vi "FlatToRichniswitch_grpc_RouteScanAdvancedOutputRequest.vi"(5 "OutputClusterType":T1, 11 "InputCluster":T3) -> (3 "OutputCluster":T1)   [LabVIEW 2021, in "NI Switch_client.lvlib"]
uses:
  NI Switch_client.lvlib
  niswitch_grpc_RouteScanAdvancedOutputRequest_scan_advanced_output_connector_enum/niswitch_grpc_RouteScanAdvancedOutputRequest_scan_advanced_output_connector_enum.lvclass
  niswitch_grpc_RouteScanAdvancedOutputRequest_scan_advanced_output_bus_line_enum/niswitch_grpc_RouteScanAdvancedOutputRequest_scan_advanced_output_bus_line_enum.lvclass
  nidevice_grpc_Session.ctl
  niswitch_grpc_RouteScanAdvancedOutputRequest.ctl
  niswitch_grpc_ScanAdvancedOutput.ctl
  nidevice_grpc_Session_Flat.ctl
  niswitch_grpc_RouteScanAdvancedOutputRequest_Flat.ctl
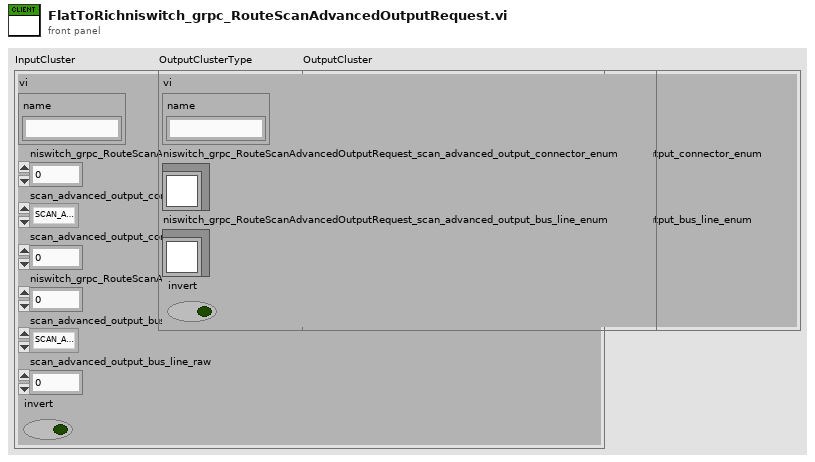
[diagram p1: front panel]
types:
  T1 = typedef "NI Switch_client.lvlib/niswitch_grpc_RouteScanAdvancedOutputRequest.ctl" = cluster{"vi":T2, "niswitch_grpc_RouteScanAdvancedOutputRequest_scan_advanced_output_connector_enum":refnum<class "niswitch_grpc_RouteScanAdvancedOutputRequest_scan_advanced_output_connector_enum.lvclass">, "niswitch_grpc_RouteScanAdvancedOutputRequest_scan_advanced_output_bus_line_enum":refnum<class "niswitch_grpc_RouteScanAdvancedOutputRequest_scan_advanced_output_bus_line_enum.lvclass">, "invert":bool}
  T2 = typedef "NI Switch_client.lvlib/nidevice_grpc_Session.ctl" = cluster{"name":string}
  T3 = typedef "NI Switch_client.lvlib/niswitch_grpc_RouteScanAdvancedOutputRequest_Flat.ctl" = cluster{"vi":T4, "niswitch_grpc_RouteScanAdvancedOutputRequest_scan_advanced_output_connector_enum_selected_index":i32, "scan_advanced_output_connector":T5, "scan_advanced_output_connector_raw":i32, "niswitch_grpc_RouteScanAdvancedOutputRequest_scan_advanced_output_bus_line_enum_selected_index":i32, "scan_advanced_output_bus_line":T5, "scan_advanced_output_bus_line_raw":i32, "invert":bool}
  T4 = typedef "NI Switch_client.lvlib/nidevice_grpc_Session_Flat.ctl" = cluster{"name":string}
  T5 = typedef "NI Switch_client.lvlib/niswitch_grpc_ScanAdvancedOutput.ctl" = enum32{"SCAN_ADVANCED_OUTPUT_NISWITCH_VAL_NONE", "SCAN_ADVANCED_OUTPUT_NISWITCH_VAL_EXTERNAL", "SCAN_ADVANCED_OUTPUT_NISWITCH_VAL_TTL0", "SCAN_ADVANCED_OUTPUT_NISWITCH_VAL_TTL1", "SCAN_ADVANCED_OUTPUT_NISWITCH_VAL_TTL2", "SCAN_ADVANCED_OUTPUT_NISWITCH_VAL_TTL3", "SCAN_ADVANCED_OUTPUT_NISWITCH_VAL_TTL4", "SCAN_ADVANCED_OUTPUT_NISWITCH_VAL_TTL5", "SCAN_ADVANCED_OUTPUT_NISWITCH_VAL_TTL6", "SCAN_ADVANCED_OUTPUT_NISWITCH_VAL_TTL7", "SCAN_ADVANCED_OUTPUT_NISWITCH_VAL_PXI_STAR", "SCAN_ADVANCED_OUTPUT_NISWITCH_VAL_REARCONNECTOR", "SCAN_ADVANCED_OUTPUT_NISWITCH_VAL_FRONTCONNECTOR", "SCAN_ADVANCED_OUTPUT_NISWITCH_VAL_REARCONNECTOR_MODULE1", "SCAN_ADVANCED_OUTPUT_NISWITCH_VAL_REARCONNECTOR_MODULE2", "SCAN_ADVANCED_OUTPUT_NISWITCH_VAL_REARCONNECTOR_MODULE3", "SCAN_ADVANCED_OUTPUT_NISWITCH_VAL_REARCONNECTOR_MODULE4", "SCAN_ADVANCED_OUTPUT_NISWITCH_VAL_REARCONNECTOR_MODULE5", "SCAN_ADVANCED_OUTPUT_NISWITCH_VAL_REARCONNECTOR_MODULE6", "SCAN_ADVANCED_OUTPUT_NISWITCH_VAL_REARCONNECTOR_MODULE7", "SCAN_ADVANCED_OUTPUT_NISWITCH_VAL_REARCONNECTOR_MODULE8", "SCAN_ADVANCED_OUTPUT_NISWITCH_VAL_REARCONNECTOR_MODULE9", "SCAN_ADVANCED_OUTPUT_NISWITCH_VAL_REARCONNECTOR_MODULE10", "SCAN_ADVANCED_OUTPUT_NISWITCH_VAL_REARCONNECTOR_MODULE11", "SCAN_ADVANCED_OUTPUT_NISWITCH_VAL_REARCONNECTOR_MODULE12", "SCAN_ADVANCED_OUTPUT_NISWITCH_VAL_FRONTCONNECTOR_MODULE1", "SCAN_ADVANCED_OUTPUT_NISWITCH_VAL_FRONTCONNECTOR_MODULE2", "SCAN_ADVANCED_OUTPUT_NISWITCH_VAL_FRONTCONNECTOR_MODULE3", "SCAN_ADVANCED_OUTPUT_NISWITCH_VAL_FRONTCONNECTOR_MODULE4", "SCAN_ADVANCED_OUTPUT_NISWITCH_VAL_FRONTCONNECTOR_MODULE5", "SCAN_ADVANCED_OUTPUT_NISWITCH_VAL_FRONTCONNECTOR_MODULE6", "SCAN_ADVANCED_OUTPUT_NISWITCH_VAL_FRONTCONNECTOR_MODULE7", "SCAN_ADVANCED_OUTPUT_NISWITCH_VAL_FRONTCONNECTOR_MODULE8", "SCAN_ADVANCED_OUTPUT_NISWITCH_VAL_FRONTCONNECTOR_MODULE9", "SCAN_ADVANCED_OUTPUT_NISWITCH_VAL_FRONTCONNECTOR_MODULE10", "SCAN_ADVANCED_OUTPUT_NISWITCH_VAL_FRONTCONNECTOR_MODULE11", "SCAN_ADVANCED_OUTPUT_NISWITCH_VAL_FRONTCONNECTOR_MODULE12"}
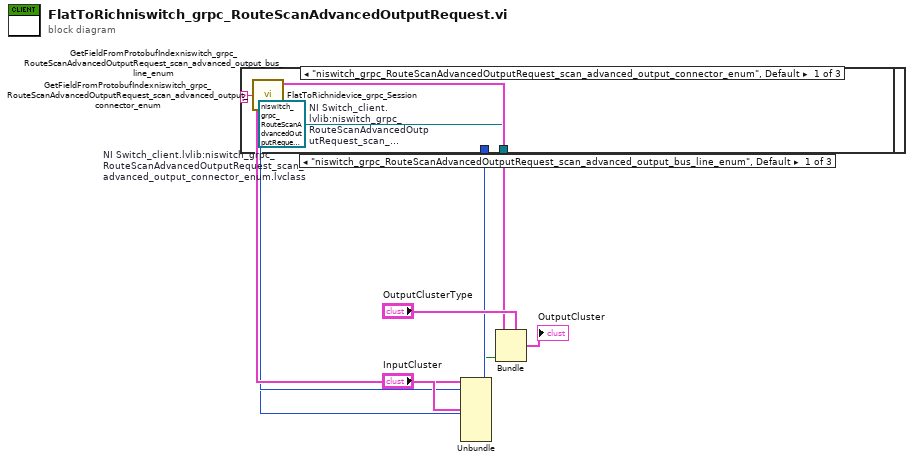
[diagram p0: block diagram]
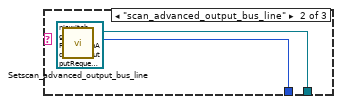
[diagram p2: hidden frame]
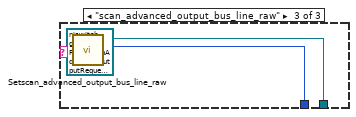
[diagram p3: hidden frame]
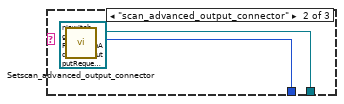
[diagram p4: hidden frame]
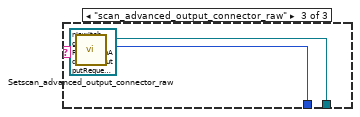
[diagram p5: hidden frame]
diagram:
  n1 = Unbundle "Unbundle"("InputCluster") -> ("vi"=w13:T4, "niswitch_grpc_RouteScanAdvancedOutputRequest_scan_advanced_output_connector_enum_selected_index"=w11:i32, "scan_advanced_output_connector"=w8:T5, "scan_advanced_output_connector_raw"=w7:i32, "niswitch_grpc_RouteScanAdvancedOutputRequest_scan_advanced_output_bus_line_enum_selected_index"=w6:i32, "scan_advanced_output_bus_line"=w3:T5, "scan_advanced_output_bus_line_raw"=w2:i32, "invert"=w1:bool)
  n2 = call "GetFieldFromProtobufIndexniswitch_grpc_RouteScanAdvancedOutputRequest_scan_advanced_output_bus_line_enum.vi"("protobuf index"=w6) -> ("oneof field name"=w5:string)
  n3 = case "niswitch_grpc_RouteScanAdvancedOutputRequest_scan_advanced_output_bus_line_enum" shown="\"niswitch_grpc_RouteScanAdvancedOutputRequest_scan_advanced_output_bus_line_enum\", Default" w5 {
    tunnel: [w17 w19 w22] -> w4
    tunnel: w3 -> [_ w20 _]
    tunnel: w2 -> [_ _ w23]
    frame "niswitch_grpc_RouteScanAdvancedOutputRequest_scan_advanced_output_bus_line_enum", Default {
      w17 = refnum<class "niswitch_grpc_RouteScanAdvancedOutputRequest_scan_advanced_output_bus_line_enum.lvclass"> refnum  # NI Switch_client.lvlib:niswitch_grpc_RouteScanAdvancedOutputRequest_scan_advanced_output_bus_line_enum.lvclass
    }
    frame "scan_advanced_output_bus_line" {
      n4 = call "Setscan_advanced_output_bus_line.vi"("Set_Val"=w20, "OneOfTemplate in"=refnum<class "niswitch_grpc_RouteScanAdvancedOutputRequest_scan_advanced_output_bus_line_enum.lvclass"> refnum) -> ("OneOfTemplate out"=w19:refnum<class "niswitch_grpc_RouteScanAdvancedOutputRequest_scan_advanced_output_bus_line_enum.lvclass">)  [unwired: 8 in, 1 out]
    }
    frame "scan_advanced_output_bus_line_raw" {
      n5 = call "Setscan_advanced_output_bus_line_raw.vi"("Set_Val"=w23, "OneOfTemplate in"=refnum<class "niswitch_grpc_RouteScanAdvancedOutputRequest_scan_advanced_output_bus_line_enum.lvclass"> refnum) -> ("OneOfTemplate out"=w22:refnum<class "niswitch_grpc_RouteScanAdvancedOutputRequest_scan_advanced_output_bus_line_enum.lvclass">)  [unwired: 8 in, 1 out]
    }
  }
  n6 = call "GetFieldFromProtobufIndexniswitch_grpc_RouteScanAdvancedOutputRequest_scan_advanced_output_connector_enum.vi"("protobuf index"=w11) -> ("oneof field name"=w10:string)
  n7 = case "niswitch_grpc_RouteScanAdvancedOutputRequest_scan_advanced_output_connector_enum" shown="\"niswitch_grpc_RouteScanAdvancedOutputRequest_scan_advanced_output_connector_enum\", Default" w10 {
    tunnel: [w24 w26 w29] -> w9
    tunnel: w8 -> [_ w27 _]
    tunnel: w7 -> [_ _ w30]
    frame "niswitch_grpc_RouteScanAdvancedOutputRequest_scan_advanced_output_connector_enum", Default {
      w24 = refnum<class "niswitch_grpc_RouteScanAdvancedOutputRequest_scan_advanced_output_connector_enum.lvclass"> refnum  # NI Switch_client.lvlib:niswitch_grpc_RouteScanAdvancedOutputRequest_scan_advanced_output_connector_enum.lvclass
    }
    frame "scan_advanced_output_connector" {
      n8 = call "Setscan_advanced_output_connector.vi"("Set_Val"=w27, "OneOfTemplate in"=refnum<class "niswitch_grpc_RouteScanAdvancedOutputRequest_scan_advanced_output_connector_enum.lvclass"> refnum) -> ("OneOfTemplate out"=w26:refnum<class "niswitch_grpc_RouteScanAdvancedOutputRequest_scan_advanced_output_connector_enum.lvclass">)  [unwired: 8 in, 1 out]
    }
    frame "scan_advanced_output_connector_raw" {
      n9 = call "Setscan_advanced_output_connector_raw.vi"("Set_Val"=w30, "OneOfTemplate in"=refnum<class "niswitch_grpc_RouteScanAdvancedOutputRequest_scan_advanced_output_connector_enum.lvclass"> refnum) -> ("OneOfTemplate out"=w29:refnum<class "niswitch_grpc_RouteScanAdvancedOutputRequest_scan_advanced_output_connector_enum.lvclass">)  [unwired: 8 in, 1 out]
    }
  }
  n10 = call "FlatToRichnidevice_grpc_Session.vi"("InputCluster"=w13) -> ("OutputCluster"=w12:T2)  [unwired: 10 in]
  n11 = Bundle "Bundle"(cluster="OutputClusterType", "vi"=w12, "niswitch_grpc_RouteScanAdvancedOutputRequest_scan_advanced_output_connector_enum"=w9, "niswitch_grpc_RouteScanAdvancedOutputRequest_scan_advanced_output_bus_line_enum"=w4, "invert"=w1) -> (→"OutputCluster":T1)
